vi "Convert version to numeric.vi"(9 "Version-String":string) -> (1 "Version-Numeric":u32)   [LabVIEW 2016, in "RT Management.lvlib"]
doc: "Converts the version string for a product to a numeric value for comparison. Examples that are handled: 7, 7.1, 7.1.1, 7.1.1f3 (and trailing zeros and a, b, c, and d as well as f builds)"
uses:
  RT Management.lvlib
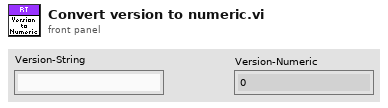
[diagram p1: front panel]
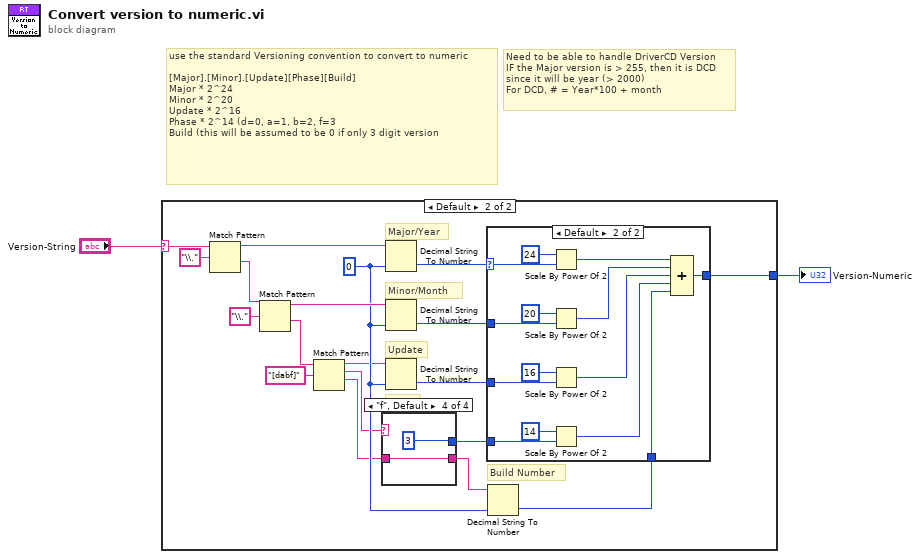
[diagram p0: block diagram]
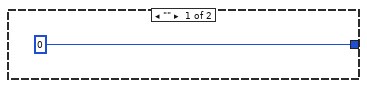
[diagram p2: hidden frame]
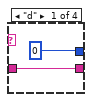
[diagram p3: hidden frame]
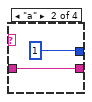
[diagram p4: hidden frame]
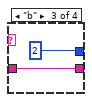
[diagram p5: hidden frame]
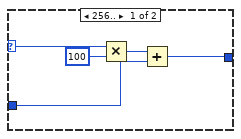
[diagram p6: hidden frame]
diagram:
  # "Need to be able to handle DriverCD Version\nIF the Major version is > 255, then it is DCD\nsince it will be year (> 2000)\nFor DCD, # = Year*100 + month"
  # "use the standard Versioning convention to convert to numeric\n\n[Major].[Minor].[Update][Phase][Build]\nMajor * 2^24\nMinor * 2^20\nUpdate * 2^16\nPhase * 2^14 (d=0, a=1, b=2, f=3\nBuild (this will be assumed to be 0 if only 3 digit version"
  n1 = case shown="Default" "Version-String" {
    selector: "Version-String" -> [_ w12]
    tunnel: [u32 0 w16] -> w1
    frame "" {
    }
    frame Default {
      w15 = u32 0 ("default (0 I32)")
      # "Phase"
      # "Update"
      # "Minor/Month"
      # "Major/Year"
      # "Build Number"
      n2 = Match Pattern(string=w12, regular expression="\\.") -> (before substring=w20:string, after substring=w19:string)  [unwired: 3 out]
      n3 = Match Pattern(string=w19, regular expression="\\.") -> (before substring=w17:string, after substring=w11:string)  [unwired: 3 out]
      n4 = Match Pattern(string=w11, regular expression="[dabf]") -> (before substring=w10:string, match substring=w7:string, after substring=w5:string)  [unwired: 2 out]
      n5 = case shown="\"f\", Default" w7 {
        tunnel: [u32 0 ("n") u32 1 ("n") u32 2 ("n") u32 3 ("n")] -> w6
        tunnel: w5 -> [w23 w25 w27 w29]
        tunnel: [w23 w25 w27 w29] -> w4
        frame "d" {
        }
        frame "a" {
        }
        frame "b" {
        }
        frame "f", Default {
        }
      }
      n6 = Decimal String To Number(string=w20, default (0L)=w15) -> (number=w8:u32)  [unwired: 2 out]
      n7 = Decimal String To Number(string=w17, default (0L)=w15) -> (number=w13:u32)  [unwired: 2 out]
      n8 = Decimal String To Number(string=w10, default (0L)=w15) -> (number=w14:u32)  [unwired: 2 out]
      n9 = Decimal String To Number(string=w4, default (0L)=w15) -> (number=w9:u32)  [unwired: 2 out]
      n10 = case shown="Default" w8 {
        selector: w8 -> [w35 w37]
        tunnel: [w31 w45] -> w16
        tunnel: w14 -> [_ w40]
        tunnel: w13 -> [w32 w39]
        tunnel: w9 -> [_ w38]
        tunnel: w6 -> [_ w36]
        frame 256.. {
          n11 = Multiply(x=w35, y=u32 100) -> (x*y=w33:u32)
          n12 = Add(x=w33, y=w32) -> (x+y=w31:u32)
        }
        frame Default {
          n13 = Scale By Power Of 2(n=24, x=w37) -> (x*2^n=w44:u32)
          n14 = Scale By Power Of 2(n=20, x=w39) -> (x*2^n=w43:u32)
          n15 = Scale By Power Of 2(n=16, x=w40) -> (x*2^n=w42:u32)
          n16 = Scale By Power Of 2(n=14, x=w36) -> (x*2^n=w41:u32)
          n17 = Compound Arithmetic op=ADD(w44, w43, w42, w41, w38) -> (w45:u32)
        }
      }
    }
  }
  "Version-Numeric" <- w1
